vi "Configure Voltage Range.vi"(7 "Voltage Range (0: Low)":i32(ring) items=["Low", "High"], 8 "error in (no error)":errorcluster, 10 "Channel (1)":string="1", 11 "VISA resource name":refnum<visa-resource-name>) -> (0 "error out":errorcluster, 3 "VISA resource name out":refnum<visa-resource-name>)   [LabVIEW 2020, in "Keysight E36300 Series.lvlib"]
doc: "Configures the voltage range."
uses:
  Keysight E36300 Series.lvlib
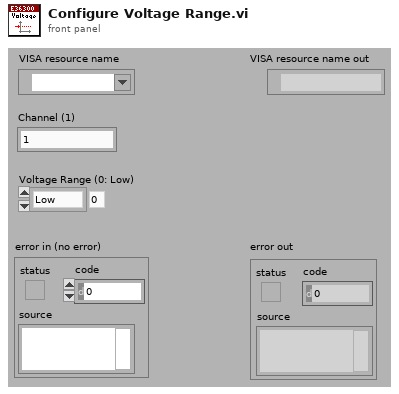
[diagram p1: front panel]
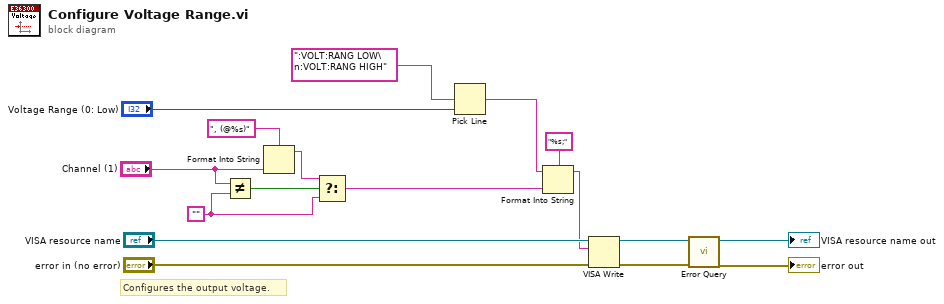
[diagram p0: block diagram]
diagram:
  w1 = ""
  # "Configures the output voltage."
  n1 = Not Equal?(x="Channel (1)", y=w1) -> (x != y?=w5:bool)
  n2 = Format Into String(format string=", (@%s)", "Channel (1)") -> (resulting string=w6:string)  [unwired: 2 in, 1 out]
  n3 = Select(t=w6, s=w5, f=w1) -> (s? t:f=w3:string)
  n4 = Pick Line(multi-line string=":VOLT:RANG LOW\n:VOLT:RANG HIGH", line index="Voltage Range (0: Low)") -> (output string=w9:string)  [unwired: 1 in]
  n5 = Format Into String(format string="%s;", initial string=w9, w3) -> (resulting string=w8:string)  [unwired: 1 in, 1 out]
  n6 = VISA Write(VISA resource name="VISA resource name", write buffer=w8, error in (no error)="error in (no error)") -> (VISA resource name out=w13:refnum<visa-resource-name>, error out=w12:errorcluster)  [unwired: 1 out]
  n7 = call "Error Query.vi"("error in (no error)"=w12, "VISA resource name"=w13) -> ("error out"=→"error out":errorcluster, "VISA resource name out"=→"VISA resource name out":refnum<visa-resource-name>)  [unwired: 6 in, 2 out]
